vi "CFU_7p1_TEAM006.vi"() -> ()   [LabVIEW 2016]
uses:
  <vilib>/express/express arith-compare/Formula/XNode/ExpressFormulaBlockNode.xnode
panel:
  out "Updated Population (Updated n)":dbl
  in  "No. of years to track":dbl
  in  "Carrying capacity (k)":dbl
  in  "Death Rate":dbl
  in  "Birth Rate":dbl
  in  "Initial Population (n)":dbl
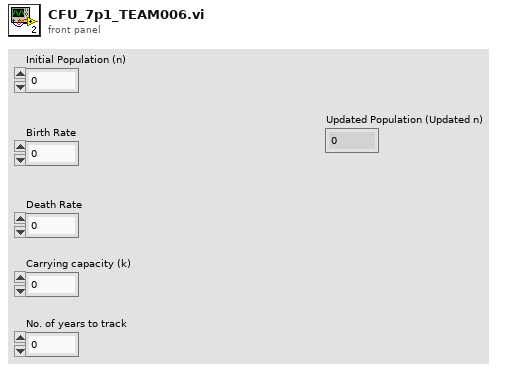
[diagram p1: front panel]
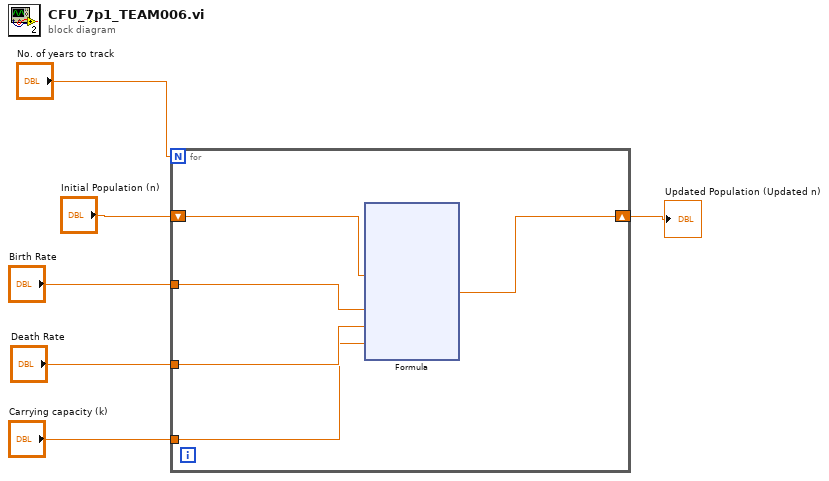
[diagram p0: block diagram]
diagram:
  n1 = for {
    N: "No. of years to track" -> [_]
    tunnel: "Birth Rate" -> [w10]
    tunnel: "Death Rate" -> [w9]
    tunnel: "Carrying capacity (k)" -> [w8]
    shift-right: [w7] -> w1
    shift-left: "Initial Population (n)" -> [w11]
    n2 = xnode "Formula"("n"=w11, "BR"=w10, "DR"=w9, "k"=w8) -> ("Result"=w7:dbl)  [unwired: 1 in, 1 out]
  }
  "Updated Population (Updated n)" <- w1
